vi "CLD 17 GUI number pad.vi"() -> ()   [LabVIEW 2020]
doc: "CLD 17\n\nThis VI uses a polling method to respond to changes in the GUI."
uses:
  CLD 17 Keypad_Typedef.ctl
panel:
  out "String":string="0"
  out "Numeric":dbl
  in  "Keypad Cluster":T1
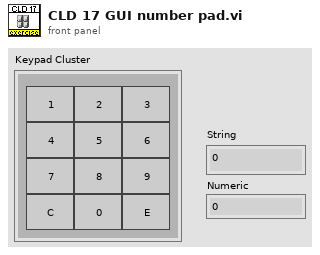
[diagram p1: front panel]
types:
  T1 = typedef "CLD 17 Keypad_Typedef.ctl" = cluster{"0":bool, "1":bool, "2":bool, "3":bool, "4":bool, "5":bool, "6":bool, "7":bool, "8":bool, "9":bool, "C":bool, "E":bool}
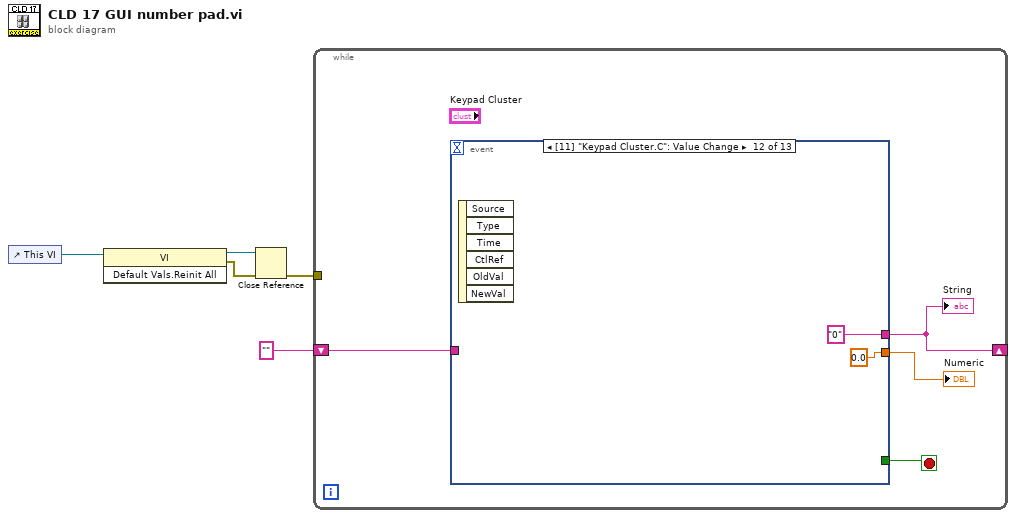
[diagram p0: block diagram]
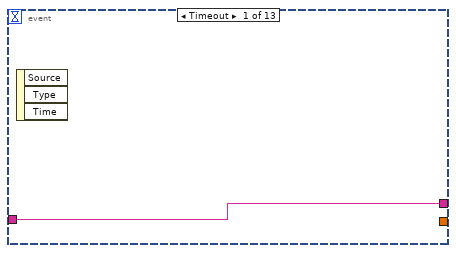
[diagram p2: hidden frame]
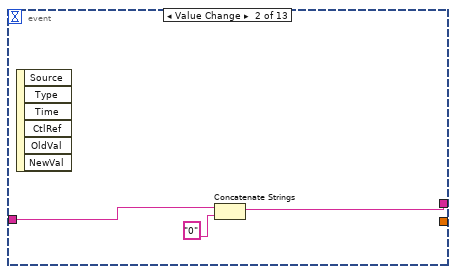
[diagram p3: hidden frame]
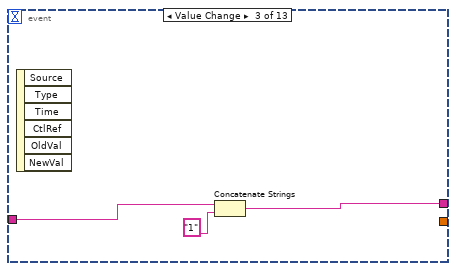
[diagram p4: hidden frame]
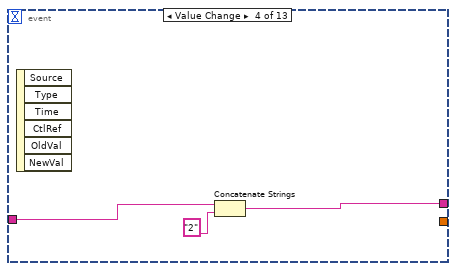
[diagram p5: hidden frame]
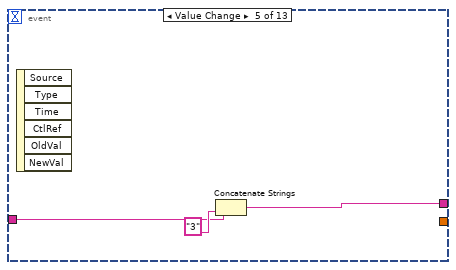
[diagram p6: hidden frame]
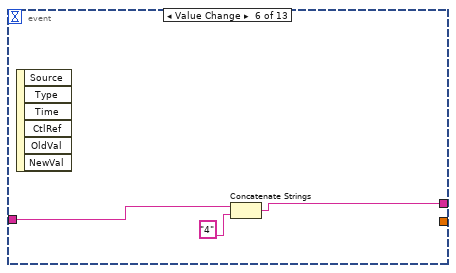
[diagram p7: hidden frame]
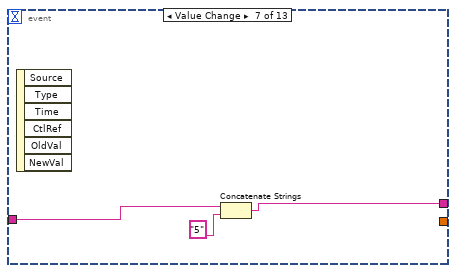
[diagram p8: hidden frame]
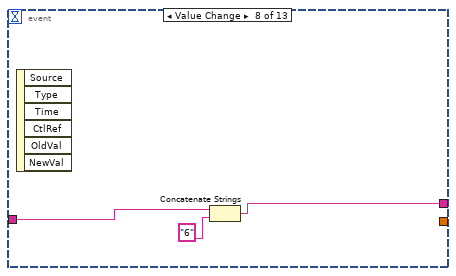
[diagram p9: hidden frame]
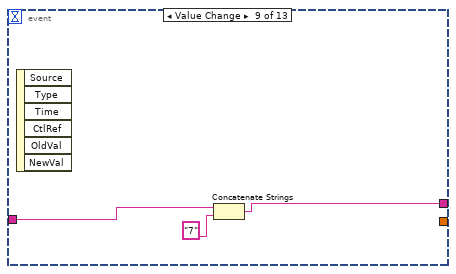
[diagram p10: hidden frame]
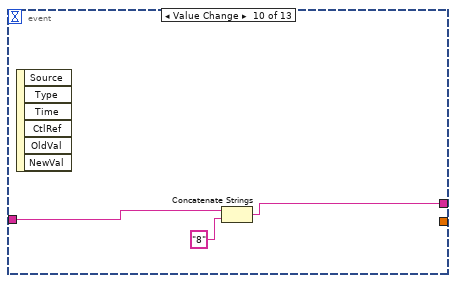
[diagram p11: hidden frame]
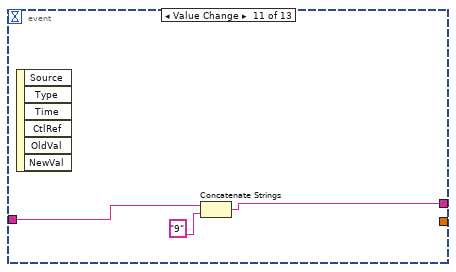
[diagram p12: hidden frame]
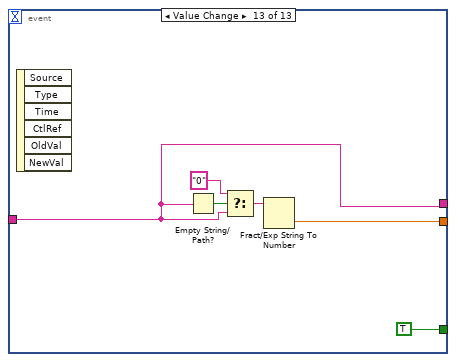
[diagram p13: hidden frame]
diagram:
  n1 = control-ref of="This VI"() -> (w3:refnum<vi>)
  n2 = invoke class="VI" method="Default Vals.Reinit All"(reference=w3) -> (reference out=w2:refnum<vi>, error out=w1:errorcluster)  [unwired: 2 in, 1 out]
  n3 = Close Reference(reference=w2, error in (no error)=w1) -> (error out=w4:errorcluster)
  n4 = while {
    shift-right: [w8] -> _
    shift-left: "" ("String") -> [w9]
    tunnel: w4 -> [_]
    stop <- w6 stop-if-true
    n5 = event shown="[11] \"Keypad Cluster.C\": Value Change" {
      selector: _ -> [_ _ _ _ _ _ _ _ _ _ _ _ _]
      dyn-events: _ -> [_ _ _ _ _ _ _ _ _ _ _ _ _]
      timeout: _ -> [_ _ _ _ _ _ _ _ _ _ _ _ _]
      tunnel: [w10 w11 w15 w18 w20 w23 w26 w29 w32 w35 w38 "0" ("String") w44] -> w8
      tunnel: w9 -> [w10 w12 w16 w19 w21 w24 w27 w30 w33 w36 w39 _ w44]
      tunnel: [_ _ _ _ _ _ _ _ _ _ _ 0.0 ("Numeric") w45] -> w7
      tunnel: [_ _ _ _ _ _ _ _ _ _ _ _ TRUE] -> w6
      event Timeout {
        n6 = event-data() -> ()  [unwired: 1 in, 3 out]
      }
      event Value Change {
        n7 = event-data() -> ()  [unwired: 1 in, 6 out]
        n8 = Concatenate Strings(w12, "0" ("string")) -> (w11:string)
      }
      event Value Change {
        n9 = event-data() -> ()  [unwired: 1 in, 6 out]
        n10 = Concatenate Strings(w16, "1" ("string")) -> (w15:string)
      }
      event Value Change {
        n11 = event-data() -> ()  [unwired: 1 in, 6 out]
        n12 = Concatenate Strings(w19, "2" ("string")) -> (w18:string)
      }
      event Value Change {
        n13 = event-data() -> ()  [unwired: 1 in, 6 out]
        n14 = Concatenate Strings(w21, "3" ("string")) -> (w20:string)
      }
      event Value Change {
        n15 = event-data() -> ()  [unwired: 1 in, 6 out]
        n16 = Concatenate Strings(w24, "4" ("string")) -> (w23:string)
      }
      event Value Change {
        n17 = event-data() -> ()  [unwired: 1 in, 6 out]
        n18 = Concatenate Strings(w27, "5" ("string")) -> (w26:string)
      }
      event Value Change {
        n19 = event-data() -> ()  [unwired: 1 in, 6 out]
        n20 = Concatenate Strings(w30, "6" ("string")) -> (w29:string)
      }
      event Value Change {
        n21 = event-data() -> ()  [unwired: 1 in, 6 out]
        n22 = Concatenate Strings(w33, "7" ("string")) -> (w32:string)
      }
      event Value Change {
        n23 = event-data() -> ()  [unwired: 1 in, 6 out]
        n24 = Concatenate Strings(w36, "8" ("string")) -> (w35:string)
      }
      event Value Change {
        n25 = event-data() -> ()  [unwired: 1 in, 6 out]
        n26 = Concatenate Strings(w39, "9" ("string")) -> (w38:string)
      }
      event Value Change {
        n27 = event-data() -> ()  [unwired: 1 in, 6 out]
      }
      event Value Change {
        n28 = event-data() -> ()  [unwired: 1 in, 6 out]
        n29 = Empty String/Path?(string/path=w44) -> (empty?=w47:bool)
        n30 = Select(t="0" ("string"), s=w47, f=w44) -> (s? t:f=w48:string)
        n31 = Fract/Exp String To Number(string=w48) -> (number=w45:dbl)  [unwired: 3 in, 1 out]
      }
    }
    "String" <- w8
    "Numeric" <- w7
  }
